vi "PH_BeamlineController.set current Value of Source Elements.vi"(0 "VI in":refnum<vi>, 5 "error in (no error)":errorcluster) -> (14 "VI out":refnum<vi>, 19 "error out":errorcluster)   [LabVIEW 2014, in "PH_BeamlineController.lvlib"]
uses:
  PH_BeamlineController.lvlib
  PH_Beamline_Chief/PH_Beamline_Chief.Section.ctl
  PH_BeamlineInformation/PH_BeamlineInformation.lvlib
  PH_Beamline_Chief/PH_Beamline_Chief.lvlib
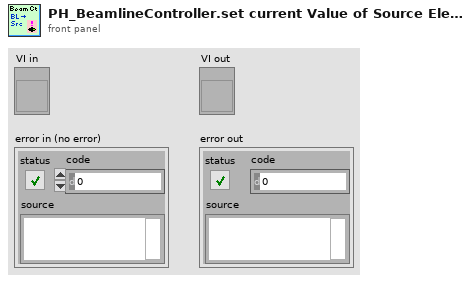
[diagram p1: front panel]
types:
  T1 = typedef "PH_BeamlineController.lvlib/PH_BeamlineController.i attribute.ctl" = cluster{"Vacuum Exp LB":cluster{"Channel":string, "Limit [mbar]":dbl, "Pressure [mbar]":dbl, "GUI Ref":refnum<vi>}, "Sources":T2[], "PA DP Targets":T4[], "Path":cluster{"Source":T3, "PA DP Target":T5, "Target":T6}, "Targets":cluster{"Name":T6, "GUI Ref":refnum<vi>, "Current State":bool, "Wanted State":bool, "Enabled":bool}[], "Status Tags":cluster{"Name":string, "Status":T7}[], "special GUI Refs":T8}
  T2 = typedef "PH_BeamlineController.lvlib/PH_BeamlineController.Source Attributes.ctl" = cluster{"Name":T3, "GUI Ref":refnum<vi>, "Current State":bool, "Wanted State":bool}
  T3 = typedef "PH_BeamlineController.lvlib/PH_BeamlineController.Sources.ctl" = enum16{"None", "YLF", "fs-Frontend", "ns-Frontend", "YLF and ns-Frontend", "fs- and ns-Frontend"}
  T4 = typedef "PH_BeamlineController.lvlib/PH_BeamlineController.PA DP Target Attributes.ctl" = cluster{"Name":T5, "GUI Ref":refnum<vi>, "Current State":bool, "Wanted State":bool, "Enabled":bool}
  T5 = typedef "PH_BeamlineController.lvlib/PH_BeamlineController.PA DP Targets.ctl" = enum16{"None", "Dump PA Delayed Beam", "Dump PA Undelayed Beam", "Dumps PA Delayed and Undelayed Beam"}
  T6 = typedef "PH_BeamlineController.lvlib/PH_BeamlineController.Targets.ctl" = enum16{"None", "PreAmp", "Dump Exp Laserlab", "Exp Laserlab", "Calorimeter", "Dump Exp Laserbay", "Exp Laserbay", "Dump Exp Z6", "Exp Z6"}
  T7 = typedef "PH_StatusHandler.lvlib/PH_StatusHandler.Status.ctl" = i16
  T8 = typedef "PH_BeamlineController.lvlib/PH_BeamlineController.special GUI Refs.ctl" = cluster{"PA-Backreflection-Meas":refnum<vi>, "fs_Synchrolock_Watch":refnum<vi>}
  T9 = cluster{"Name":T6, "GUI Ref":refnum<vi>, "Current State":bool, "Wanted State":bool, "Enabled":bool}[]
  T10 = typedef "PH_Beamline_Chief.lvlib/PH_Beamline_Chief.Section.ctl" = enum16{"None", "YLF", "fs", "fs-YLF", "ns", "PA-Input", "PA-Undelay", "PA-Delay", "PA-before-Bypass", "PA", "PA-Bypass", "PA-Exit", "PA-LL", "LL", "PA-MA", "MA-Exit", "MA-Z6", "Z6", "MA-LB", "LB-TB2", "LB-TB3"}
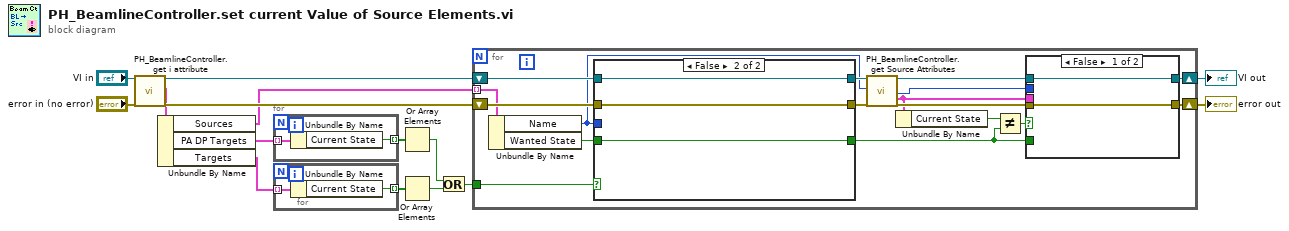
[diagram p0: block diagram]
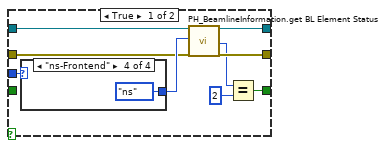
[diagram p2: hidden frame]
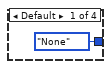
[diagram p3: hidden frame]
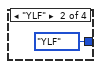
[diagram p4: hidden frame]
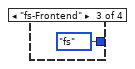
[diagram p5: hidden frame]
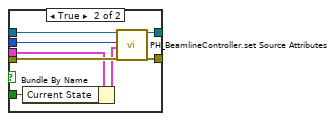
[diagram p6: hidden frame]
diagram:
  n1 = call "PH_BeamlineController.get i attribute.vi"("i ref in"="VI in", "error in (no error)"="error in (no error)") -> ("i ref out"=w13:refnum<vi>, "i attribute"=w14:T1, "error out"=w15:errorcluster)  [unwired: 15 in]
  n2 = Unbundle By Name(w14) -> ("Sources"=w10:T2[], "PA DP Targets"=w7:T4[], "Targets"=w6:T9)
  n3 = for {
    tunnel: w7 -> [w17] mode=indexing
    tunnel: [w16] -> w5 mode=indexing
    n4 = Unbundle By Name(w17) -> ("Current State"=w16:bool)
  }
  n5 = for {
    tunnel: w6 -> [w19] mode=indexing
    tunnel: [w18] -> w4 mode=indexing
    n6 = Unbundle By Name(w19) -> ("Current State"=w18:bool)
  }
  n7 = Or Array Elements(Boolean array=w5) -> (logical OR=w3:bool)
  n8 = Or Array Elements(Boolean array=w4) -> (logical OR=w2:bool)
  n9 = Or(x=w3, y=w2) -> (x .or. y?=w1:bool)
  n10 = for {
    shift-right: [w35] -> w12
    shift-left: w15 -> [w25]
    shift-right: [w33] -> w11
    shift-left: w13 -> [w22]
    tunnel: w10 -> [w23] mode=indexing
    tunnel: w1 -> [w24]
    n11 = Unbundle By Name(w23) -> ("Name"=w21:T3, "Wanted State"=w20:bool)
    n12 = case shown="False" w24 {
      tunnel: w22 -> [w45 w52]
      tunnel: [w44 w52] -> w28
      tunnel: [w43 w51] -> w27
      tunnel: [w39 w50] -> w26
      tunnel: w25 -> [w38 w51]
      tunnel: w21 -> [w37 _]
      tunnel: w20 -> [_ w50]
      frame True {
        n13 = case shown="\"ns-Frontend\"" w37 {
          tunnel: [PH_Beamline_Chief.Section."None" ("Beamline Element") PH_Beamline_Chief.Section."YLF" ("Beamline Element") PH_Beamline_Chief.Section."fs" ("Beamline Element") PH_Beamline_Chief.Section."ns" ("Beamline Element")] -> w42
          frame Default {
          }
          frame "YLF" {
          }
          frame "fs-Frontend" {
          }
          frame "ns-Frontend" {
          }
        }
        n14 = call "PH_BeamlineInformation.get BL Element Status.vi"("VI in"=w45, "Beamline Element"=w42, "error in (no error)"=w38) -> ("VI out"=w44:refnum<vi>, "Status"=w41:i32, "error out"=w43:errorcluster)  [unwired: 14 in]
        n15 = Equal?(x=w41, y=2) -> (x = y?=w39:bool)
      }
      frame False {
      }
    }
    n16 = call "PH_BeamlineController.get Source Attributes.vi"("VI in"=w28, "Source"=w21, "error in (no error)"=w27) -> ("VI out"=w34:refnum<vi>, "Source Index"=w32:i32, "Source Attributes"=w31:T2, "error out"=w36:errorcluster)  [unwired: 13 in]
    n17 = Unbundle By Name(w31) -> ("Current State"=w30:bool)
    n18 = Not Equal?(x=w30, y=w26) -> (x != y?=w29:bool)
    n19 = case shown="False" w29 {
      tunnel: w36 -> [w53 w62]
      tunnel: [w53 w61] -> w35
      tunnel: w34 -> [w54 w60]
      tunnel: [w54 w59] -> w33
      tunnel: w32 -> [_ w58]
      tunnel: w31 -> [_ w56]
      tunnel: w26 -> [_ w55]
      frame False {
      }
      frame True {
        n20 = Bundle By Name(cluster=w56, "Current State"=w55) -> (w57:T2)
        n21 = call "PH_BeamlineController.set Source Attributes.vi"("VI in"=w60, "Source Index"=w58, "Changed Source Attributes"=w57, "error in (no error)"=w62) -> ("VI out"=w59:refnum<vi>, "error out"=w61:errorcluster)  [unwired: 14 in]
      }
    }
  }
  "VI out" <- w11
  "error out" <- w12
